vi "Data Counts.vi"(8 "error in (no error)":errorcluster, 10 "Data":dbl[](array[numeric]), 11 "Initialize":bool) -> (0 "error out":errorcluster, 2 "Data Points":i32)   [LabVIEW 2015]
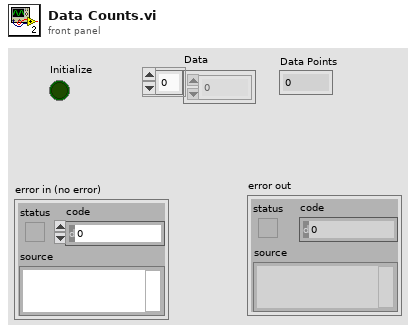
[diagram p1: front panel]
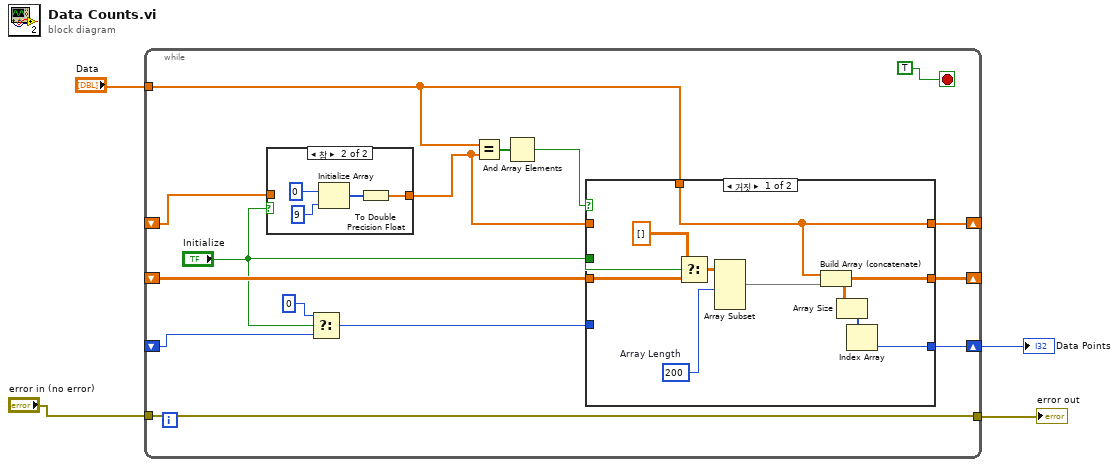
[diagram p0: block diagram]
diagram:
  n1 = while {
    tunnel: "error in (no error)" -> [w18]
    tunnel: [w18] -> w3
    shift-right: [w17] -> _
    shift-left: _ -> [w15]
    tunnel: "Data" -> [w13]
    shift-right: [w16] -> w1
    shift-left: _ -> [w9]
    shift-right: [w7] -> _
    shift-left: _ -> [w6]
    stop <- TRUE stop-if-true
    n2 = case shown="참" "Initialize" {
      tunnel: [w33 w34] -> w5
      tunnel: w6 -> [w33 _]
      frame False {
      }
      frame True {
        n3 = Initialize Array(u16 0 ("element"), 9 ("dimension size")) -> (w35:u16[])
        n4 = To Double Precision Float(number=w35) -> (double precision float=w34:dbl[])
      }
    }
    n5 = Select(t=0, s="Initialize", f=w9) -> (s? t:f=w8:i32)
    n6 = Equal?(x=w13, y=w5) -> (x = y?=w14:bool[])
    n7 = And Array Elements(Boolean array=w14) -> (logical AND=w12:bool)
    n8 = case shown="거짓" w12 {
      tunnel: [w24 w31] -> w17
      tunnel: [w23 w32] -> w16
      tunnel: "Initialize" -> [w22 _]
      tunnel: w15 -> [w21 w31]
      tunnel: w13 -> [w20 _]
      tunnel: w8 -> [_ w32]
      tunnel: [w20 w30] -> w7
      tunnel: w5 -> [_ w30]
      frame False {
        w26 = 200  # Array Length
        n9 = Select(t=dbl[][] [], s=w22, f=w21) -> (s? t:f=w27:dbl[][])
        n10 = Array Subset(array=w27, length (row)=w26) -> (w25:dbl[][])  [unwired: 3 in]
        n11 = Build Array (concatenate)(w20, w25) -> (w24:dbl[][])
        n12 = Array Size(array=w24) -> (size(s)=w29:i32[])
        n13 = Index Array(array=w29) -> (element=w23:i32)  [unwired: 1 in]
      }
      frame True {
      }
    }
  }
  "Data Points" <- w1
  "error out" <- w3
